vi "Labview6_1.vi"() -> ()   [LabVIEW 2016]
panel:
  out "Third Row Fifth Column":dbl
  in  "Rows":i32
  in  "Columns":i32
  out "Second Column":dbl[](array[numeric])
  out "Third Row":dbl[](array[numeric])
  out "Array":dbl[][](array[numeric])
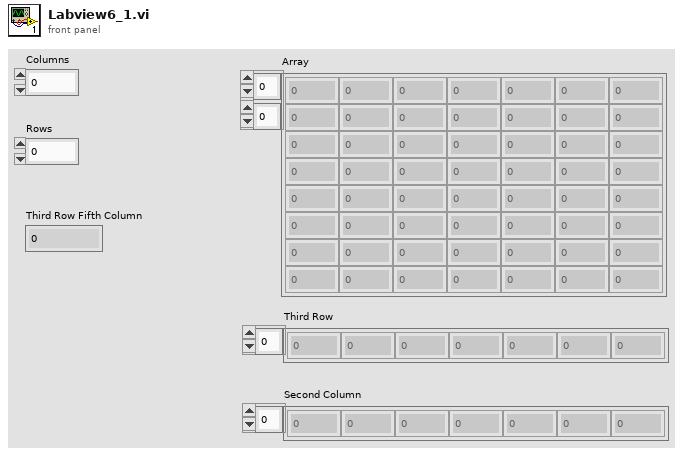
[diagram p1: front panel]
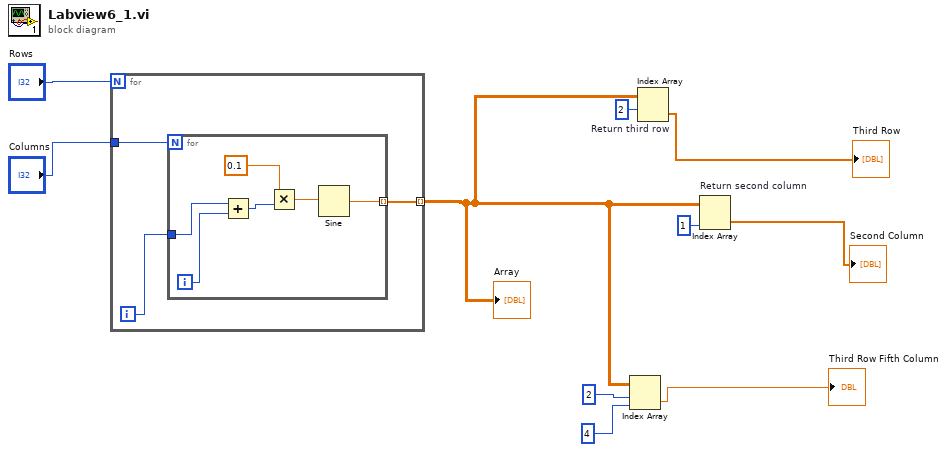
[diagram p0: block diagram]
diagram:
  n1 = for {
    N: "Rows" -> [_]
    tunnel: "Columns" -> [w13]
    tunnel: [w11] -> w2 mode=indexing
    i -> [w12]
    n2 = for {
      N: w13 -> [_]
      tunnel: w12 -> [w19]
      tunnel: [w15] -> w11 mode=indexing
      i -> [w18]
      n3 = Add(x=w19, y=w18) -> (x+y=w17:i32)
      n4 = Multiply(x=0.1, y=w17) -> (x*y=w16:dbl)
      n5 = Sine(x=w16) -> (sin(x)=w15:dbl)
    }
  }
  "Array" <- w2
  n6 = Index Array(array=w2, index (row)=2, index (col)=4 ("disabled index (col)")) -> (element=→"Third Row Fifth Column":dbl)
  n7 = Index Array "Return third row"(array=w2, index (row)=2) -> (element=→"Third Row":dbl[])  [unwired: 1 in]
  n8 = Index Array "Return second column"(array=w2, index (col)=1 ("disabled index (col)")) -> (element=→"Second Column":dbl[])  [unwired: 1 in]
